vi "Set HSE module.vi"(8 "error in (no error)":errorcluster, 10 "HSE module":bool, 11 "Library in":refnum<class "Library.lvclass">) -> (0 "error out":errorcluster, 3 "Library out":refnum<class "Library.lvclass">)   [LabVIEW 2020, in "Panther Dashboard.lvlib" / "Library.lvclass"]
uses:
  Library.lvclass
  Library.lvclass/Library.ctl
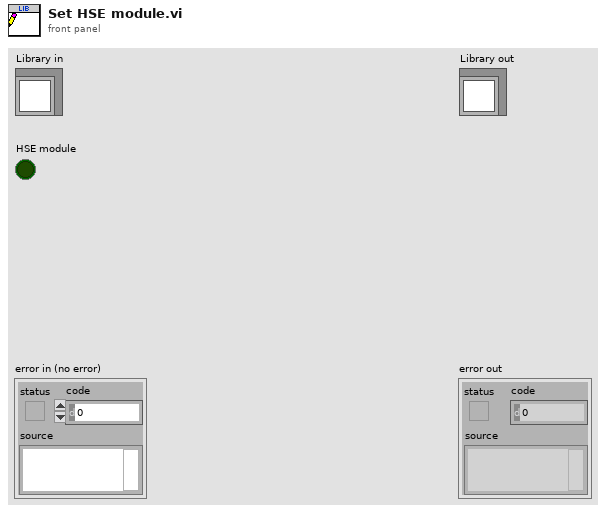
[diagram p1: front panel]
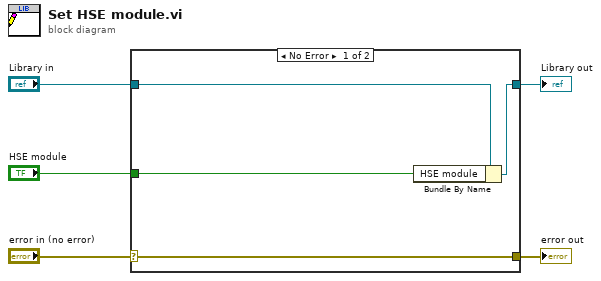
[diagram p0: block diagram]
diagram:
  n1 = case shown="No Error" "error in (no error)" {
    selector: "error in (no error)" -> [w9 w10]
    tunnel: [w9 w10] -> w4
    tunnel: [w7 w11] -> w2
    tunnel: "Library in" -> [w8 w11]
    tunnel: "HSE module" -> [w6 _]
    frame No Error {
      n2 = Bundle By Name(cluster=w8, "HSE module"=w6) -> (w7:refnum<class "Library.lvclass">)
    }
    frame Error {
    }
  }
  "error out" <- w4
  "Library out" <- w2
